vi "Read last completed stack.vi"(8 "error in (no error)":errorcluster, 10 "File name":path, 11 "Tomo in":refnum<class "Tomo.lvclass">) -> (0 "error out":errorcluster, 2 "Last completed stack":u16, 3 "Tomo out":refnum<class "Tomo.lvclass">)   [LabVIEW 2012, in "Tomo.lvclass"]
uses:
  Tomo.lvclass
  <vilib>/Utility/file.llb/Read From Spreadsheet File (I64).vi
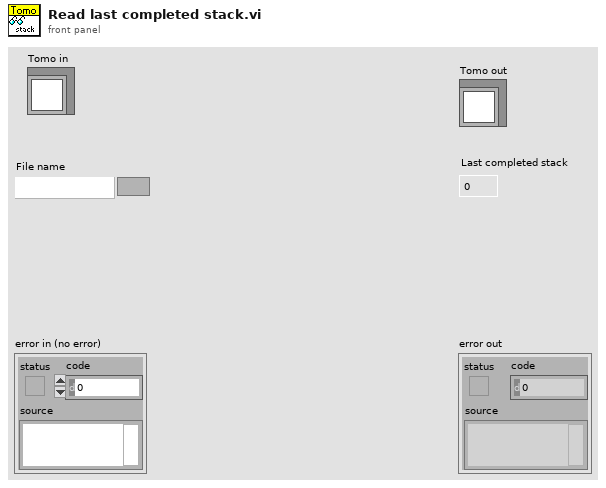
[diagram p1: front panel]
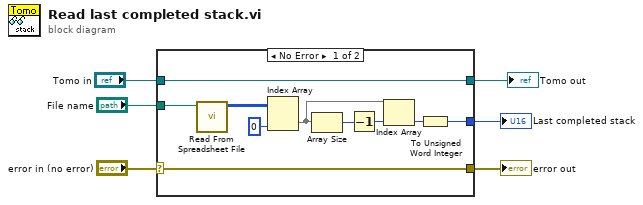
[diagram p0: block diagram]
diagram:
  n1 = case shown="No Error" "error in (no error)" {
    selector: "error in (no error)" -> [w15 w18]
    tunnel: [w15 w18] -> w5
    tunnel: [w16 w17] -> w1
    tunnel: "Tomo in" -> [w16 w17]
    tunnel: "File name" -> [w14 _]
    tunnel: [w7 _] -> w3
    frame No Error {
      n2 = call-poly <vilib>:"Read From Spreadsheet File.vi"("file path (dialog if empty)"=w14) -> ("all rows"=w13:i64[][])  [unwired: 6 in, 4 out]
      n3 = Index Array(array=w13, index (col)=0 ("index")) -> (element=w11:i64[])  [unwired: 1 in]
      n4 = Array Size(array=w11) -> (size(s)=w10:i32)
      n5 = Decrement(x=w10) -> (x-1=w9:i32)
      n6 = Index Array(array=w11, index=w9) -> (element=w8:i64)
      n7 = To Unsigned Word Integer(number=w8) -> (unsigned 16bit integer=w7:u16)
    }
    frame Error {
    }
  }
  "error out" <- w5
  "Last completed stack" <- w3
  "Tomo out" <- w1
